vi "SmartMotor Write.vi"(0 "VISA resource IN":refnum<visa-resource-name>, 1 "Motor Number":i16, 2 "Motor Command Array":string[](array[string]), 3 "Error In":errorcluster, 4 "Wait Between Writes (ms)":u32) -> (6 "VISA resource OUT":refnum<visa-resource-name>, 7 "Motor Number OUT":i16, 9 "Error Out":errorcluster)   [LabVIEW 2017, in "SmartMotor.lvclass"]
uses:
  SmartMotor.lvclass
  <vilib>/Instr/_visa.llb/VISA Flush IO Buffer Mask.ctl
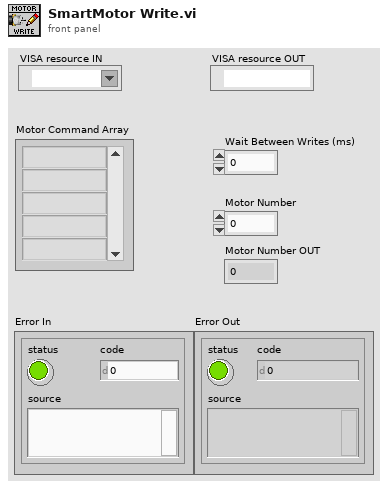
[diagram p1: front panel]
types:
  T1 = typedef "VISA Flush IO Buffer Mask.ctl" = u16
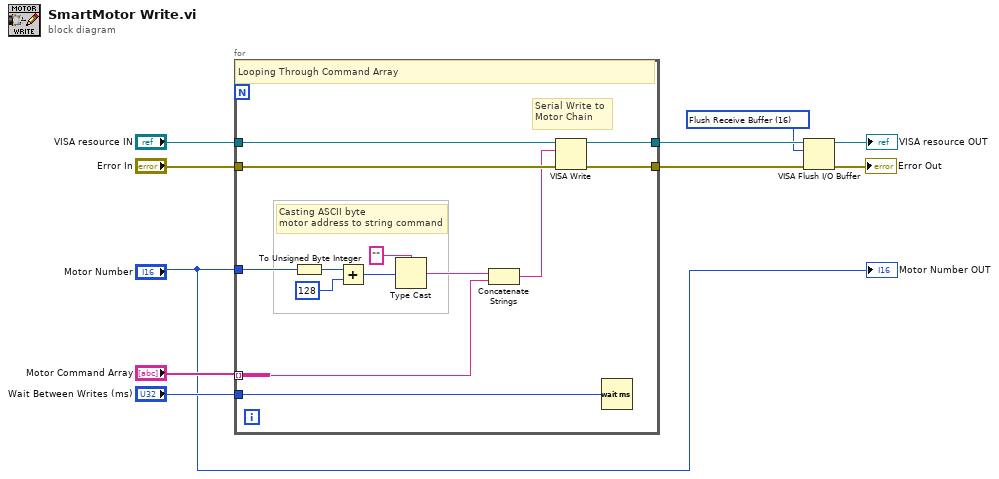
[diagram p0: block diagram]
diagram:
  w2 = T1 16 items=["Flush Receive Buffer"=16, "Write Transmit Buffer to Device"=32, "Flush Receive Buffer (No I/O)"=64, "Flush Transmit Buffer"=128] ("Mask")
  n1 = for {
    tunnel: "VISA resource IN" -> [w23]
    tunnel: [w14] -> w6
    tunnel: "Error In" -> [w22]
    tunnel: [w13] -> w3
    tunnel: "Motor Command Array" -> [w20] mode=indexing
    tunnel: "Motor Number" -> [w11]
    tunnel: "Wait Between Writes (ms)" -> [w15]
    # "Casting ASCII byte\nmotor address to string command"
    # "Serial Write to \nMotor Chain"
    # "Looping Through Command Array"
    n2 = To Unsigned Byte Integer(number=w11) -> (unsigned 8bit integer=w12:u8)
    n3 = Add(x=w12, y=u8 128) -> (x+y=w16:u8)
    n4 = Type Cast(type="", x=w16) -> (*(type *) &x=w17:string)
    n5 = Concatenate Strings(w17, w20) -> (w19:string)
    n6 = VISA Write(VISA resource name=w23, write buffer=w19, error in (no error)=w22) -> (VISA resource name out=w14:refnum<visa-resource-name>, error out=w13:errorcluster)  [unwired: 1 out]
    n7 = Wait (ms)(milliseconds to wait=w15) -> ()  [unwired: 1 out]
  }
  n8 = VISA Flush I/O Buffer(VISA resource name=w6, mask (16)=w2, error in (no error)=w3) -> (VISA resource name out=→"VISA resource OUT":refnum<visa-resource-name>, error out=→"Error Out":errorcluster)
  "Motor Number OUT" <- "Motor Number"
